vi "string2cmds_v1.vi"(7 "numCmds":i32=11, 11 "input string":string) -> (3 "output cmds":sgl[](array[numeric]))   [LabVIEW 2016]
panel:
  # ">>>"
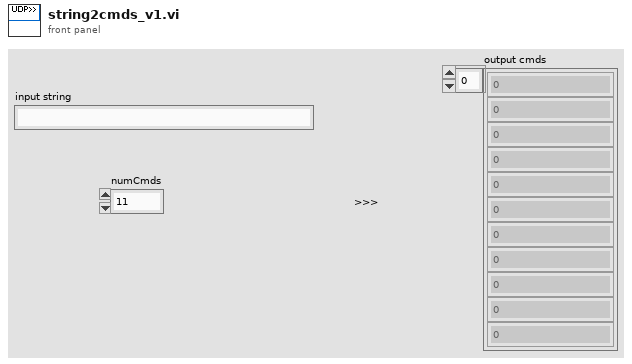
[diagram p1: front panel]
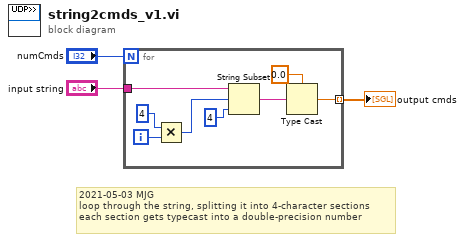
[diagram p0: block diagram]
diagram:
  # "2021-05-03 MJG\nloop through the string, splitting it into 4-character sections\neach section gets typecast into a double-precision number"
  n1 = for {
    N: "numCmds" -> [_]
    tunnel: "input string" -> [w7]
    tunnel: [w4] -> w3 mode=indexing
    i -> [w10]
    n2 = Multiply(x=4, y=w10) -> (x*y=w8:i32)
    n3 = String Subset(string=w7, offset (0)=w8, length (rest)=4 ("offset (0)")) -> (substring=w6:string)
    n4 = Type Cast(type=sgl 0.0, x=w6) -> (*(type *) &x=w4:sgl)
  }
  "output cmds" <- w3
